vi "SpreadsheetString_No_Carrage_Return_StringArray.vi"(1 "Deliminator":string="\t", 2 "Array":string[](array[string])=["", "", "", "", "", "", "", "", "", "", "", "", "", "", "", "", "", "", "", "", "", "", "", "", "", "", "", "", "", "", "", ""], 3 "Format String":string="%d") -> (0 "spreadsheet string":string="0\t0\t0\t0\t0\t1\t0\t0\t0\t0\t0\t0\t0\t0\t0\t0\t0\t0\t0\t0\t0\t0\t0\t0\t0\t0\t0\t0\t0\t0\t0\t0")   [LabVIEW 2012, in "SubVIs.lvlib"]
uses:
  SubVIs.lvlib
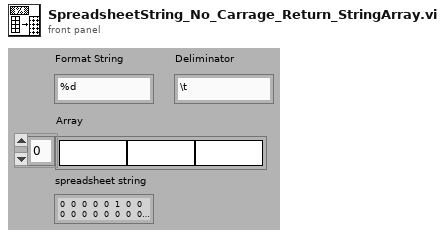
[diagram p1: front panel]
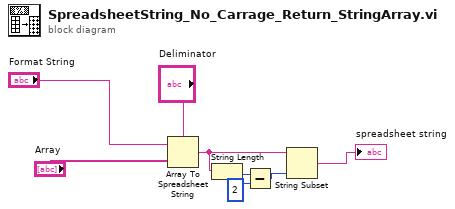
[diagram p0: block diagram]
diagram:
  n1 = Array To Spreadsheet String(delimiter (Tab)="Deliminator", array="Array", 3:"Format String") -> (spreadsheet string=w6:string)
  n2 = String Length(string=w6) -> (length=w3:i32)
  n3 = Subtract(x=w3, y=2) -> (x-y=w2:i32)
  n4 = String Subset(string=w6, length (rest)=w2) -> (substring=→"spreadsheet string":string)  [unwired: 1 out]
